vi "Msg Logger.vi"(6 "Read Error":errorcluster, 8 "Send Error":errorcluster, 9 "Recieved Packet":T1={"Packet Signature"="", "Sequence Number"=0, "Command"=enum."Get Info", "Data Message Size"=0, "Data Message Size"="", "Data Message"="", "Error Message Size"=0, "Error Message Size"="", "Error Message"="", "Checksum"=0, "Error Message"={"status"=FALSE, "code"=0, "source"=""}, "Command ID"=""}, 10 "Sent Packet":T1={"Packet Signature"="", "Sequence Number"=0, "Command"=enum."Get Info", "Data Message Size"=0, "Data Message Size"="", "Data Message"="", "Error Message Size"=0, "Error Message Size"="", "Error Message"="", "Checksum"=0, "Error Message"={"status"=FALSE, "code"=0, "source"=""}, "Command ID"=""}) -> ()   [LabVIEW 2015]
uses:
  Type/TCP Packet Info.ctl
  Type/_RT Command.ctl
panel:
  out "Msgs":string
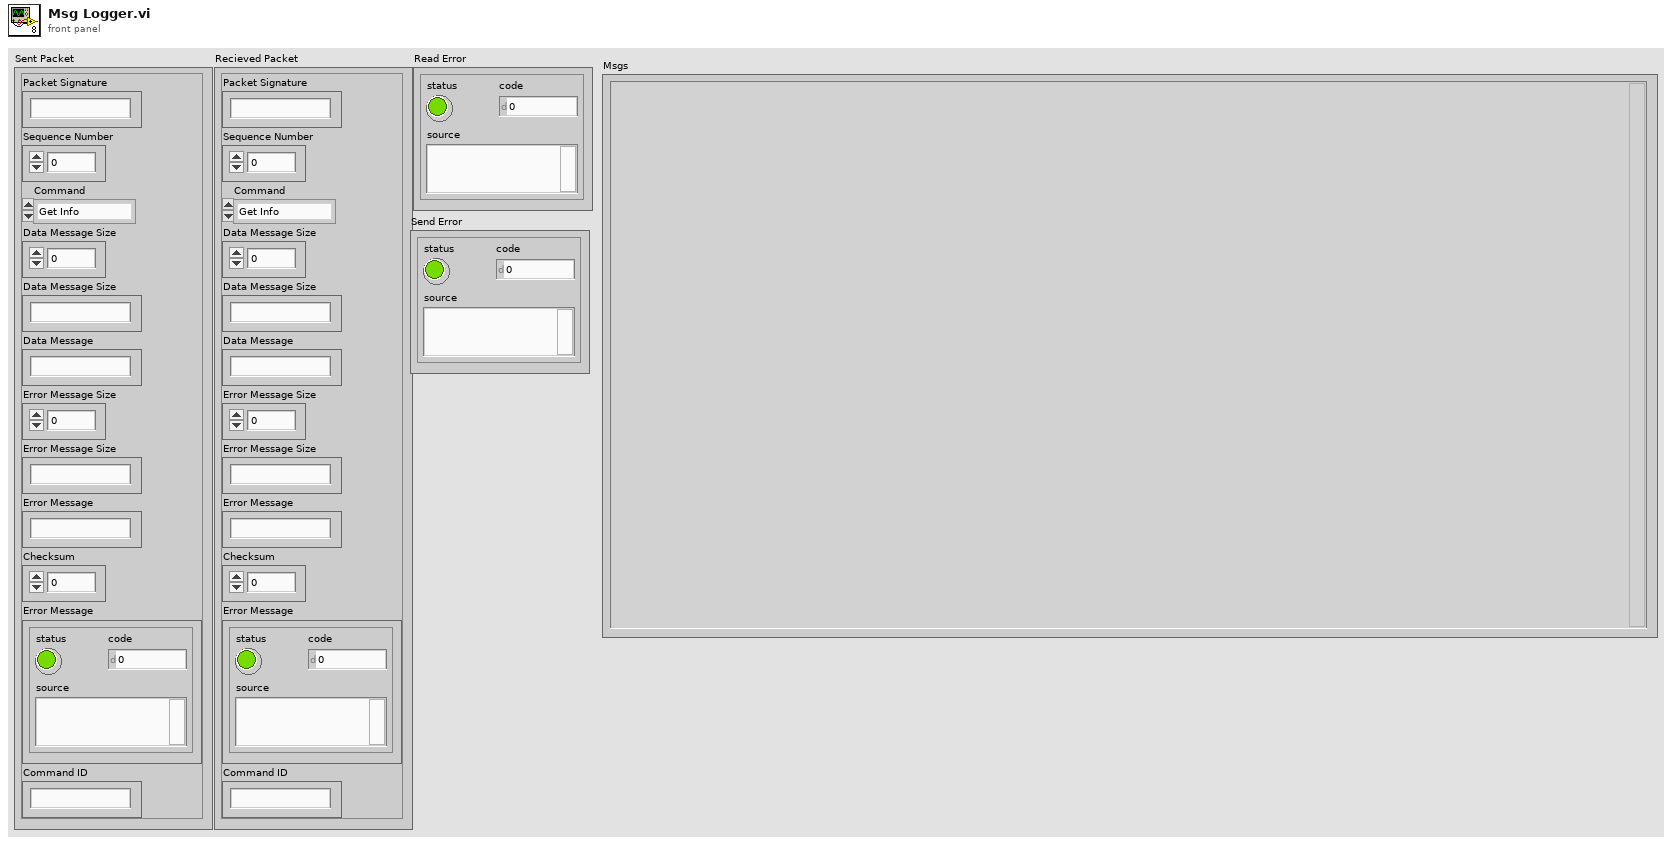
[diagram p1: front panel]
types:
  T1 = typedef "TCP Packet Info.ctl" = cluster{"Packet Signature":string, "Sequence Number":i32, "Command":T2, "Data Message Size":u32, "Data Message Size":string, "Data Message":string, "Error Message Size":u32, "Error Message Size":string, "Error Message":string, "Checksum":u32, "Error Message":errorcluster, "Command ID":string}
  T2 = typedef "_RT Command.ctl" = enum16{"xml Start Run", "xml Start Actual Run", "xml Stop Run", "xml Runtime Update", "xml Get Status", "xml Get Table", "xml Set Table", "xml Get Configuration", "xml System Status", "xml Set LC Input Logic", "xml Get Data", "xml Get Info", "Start", "StartActualRun", "Stop", "Runtime Update", "Get Data", "Get Info", "Get Status", "Get Param", "Get Config", "Get Table", "Read ADC", "Set Oscillator", "Update Config", "Update Table", "Set All Pol", "Set Pol and DC", "Set Max Mass", "Toggle RP", "Toggle EL", "Set PIC", "Initialize Turbo", "Send Turbo Comm", "Close Turbo", "P1", "P2", "P3", "Send Serial", "Set LC Out", "Get LC In", "Read VAC", "Test Table", "Toggle Power", "Get Startup", "Set Startup", "Get ADC Table", "Set ADC Table", "Get Brief Status", "Get Detail Status", "Auxiliary Update", "Set CC Logics", "Set CC Input Logics", "Ignore Error", "invalid"}
  T3 = enum32{"invalid app kind", "Development System", "Run Time System", "Student Edition", "Embedded LabVIEW", "Evaluation", "Custom"}
  T4 = enum32{"Invalid", "Standard", "Closed", "Hidden", "Minimized", "Maximized"}
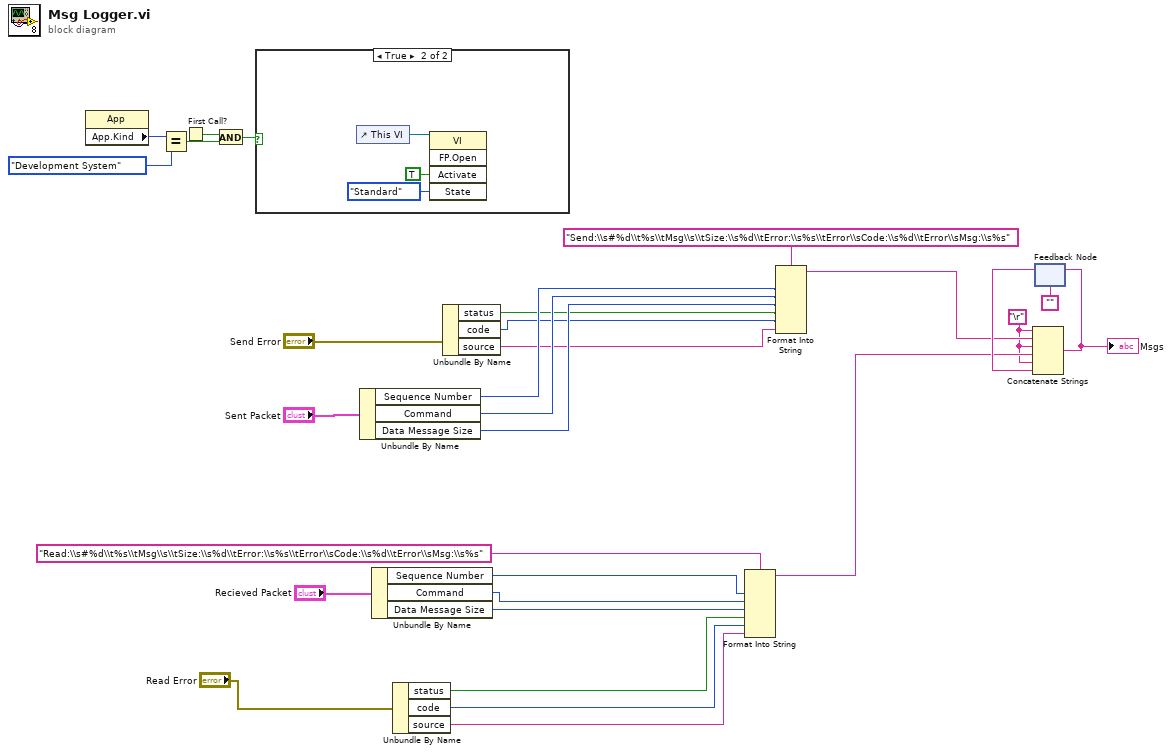
[diagram p0: block diagram]
diagram:
  w6 = "\r"
  n1 = property class="App"() -> ("App.Kind"=w5:T3)  [unwired: 2 in, 2 out]
  n2 = Equal?(x=w5, y=T3."Development System" ("Application:Kind")) -> (x = y?=w1:bool)
  n3 = First Call?() -> (First Call?: T/F=w3:bool)
  n4 = And(x=w3, y=w1) -> (x .and. y?=w2:bool)
  n5 = case shown="True" w2 {
    frame False {
    }
    frame True {
      n6 = control-ref of="This VI"() -> (w30:refnum<vi>)
      n7 = invoke class="VI" method="FP.Open"(reference=w30, "Activate"=TRUE ("Activate?"), "State"=T4."Standard") -> ()  [unwired: 2 in, 5 out]
    }
  }
  n8 = Unbundle By Name("Sent Packet") -> ("Sequence Number"=w22:i32, "Command"=w21:T2, "Data Message Size"=w20:u32)
  n9 = Unbundle By Name("Recieved Packet") -> ("Sequence Number"=w11:i32, "Command"=w16:T2, "Data Message Size"=w12:u32)
  n10 = Unbundle By Name("Read Error") -> ("status"=w15:bool, "code"=w13:i32, "source"=w14:string)
  n11 = Unbundle By Name("Send Error") -> ("status"=w19:bool, "code"=w18:i32, "source"=w17:string)
  n12 = Format Into String(format string="Read:\\s#%d\\t%s\\tMsg\\s\\tSize:\\s%d\\tError:\\s%s\\tError\\sCode:\\s%d\\tError\\sMsg:\\s%s", w11, w16, w12, w15, w13, w14) -> (resulting string=w7:string)  [unwired: 2 in, 1 out]
  n13 = Format Into String(format string="Send:\\s#%d\\t%s\\tMsg\\s\\tSize:\\s%d\\tError:\\s%s\\tError\\sCode:\\s%d\\tError\\sMsg:\\s%s", w22, w21, w20, w19, w18, w17) -> (resulting string=w25:string)  [unwired: 2 in, 1 out]
  n14 = feedback #1("") -> (w28:string)
  n15 = Concatenate Strings(w6, w25, w6, w7, w6, w28) -> (w27:string)
  "Msgs" <- w27
  n16 = feedback-in #1(w27) -> ()
